vi "Jeremy Example.vi"() -> ()   [LabVIEW 2016]
panel:
  out "Time Stamp":timestamp
  out "Waveform Graph":dbl[](graph)
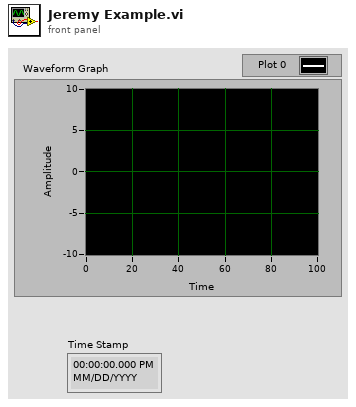
[diagram p1: front panel]
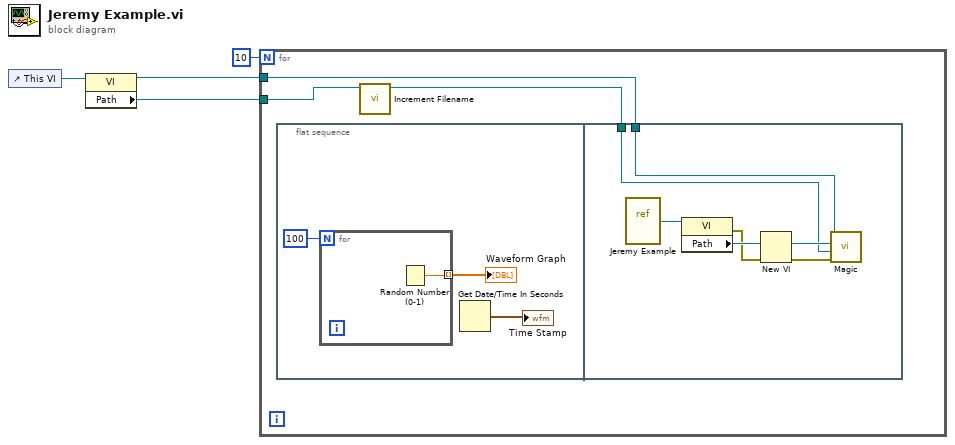
[diagram p0: block diagram]
diagram:
  n1 = control-ref of="This VI"() -> (w3:refnum<vi>)
  n2 = property class="VI"(reference=w3) -> (reference out=w1:refnum<vi>, "Path"=w2:path)  [unwired: 1 in, 1 out]
  n3 = for {
    N: 10 -> [_]
    tunnel: w2 -> [w7]
    tunnel: w1 -> [w6]
    n4 = flat-sequence {
      tunnel: w6 -> [w15]
      tunnel: w5 -> [w14]
      frame #0 {
        n5 = for {
          N: 100 -> [_]
          tunnel: [w11] -> w9 mode=indexing
          n6 = Random Number (0-1)() -> (number: 0 to 1=w11:dbl)
        }
        "Waveform Graph" <- w9
        n7 = Get Date/Time In Seconds() -> (seconds since 1Jan1904=→"Time Stamp":timestamp)
      }
      frame #1 {
        n8 = vi-ref "Jeremy Example.vi"() -> (w18:refnum<vi>)
        n9 = property class="VI"(reference=w18) -> (error out=w12:errorcluster, "Path"=w17:path)  [unwired: 1 in, 1 out]
        n10 = New VI(8:w12, 10:w17) -> (0:w13:errorcluster, 3:w16:refnum<vi>)  [unwired: 5 in]
        n11 = call "Magic.vi"("error in"=w13, "Path"=w14, "Visualize VI Ref"=w16, "Parent VI"=w15) -> ()  [unwired: 7 in, 1 out]
      }
    }
    n12 = call <userlib>:"Increment Filename.vi"("path"=w7) -> ("modified path"=w5:path)  [unwired: 9 in, 1 out]
  }
